vi "save_to_logfile.vi"(0 "file":string, 1 "header_data":string, 3 "to logfile":string[](array[string]), 4 "SAVE":bool, 6 "path":path) -> (10 "writing":bool, 18 "bytes":i64=2275764 format="%.1p")   [LabVIEW 2017, in "ZBOX_IS.lvlib"]
uses:
  ZBOX_IS.lvlib
panel:
  in  "write rate, s":dbl=1.0 min=0.1 max=10.0 step=0.1 format="%#_13g"
  out "to collect":i32=1500
  in  "clear":bool
  out "t write":dbl=3547614984.042773
  in  "DATA RATE, s":dbl=0.001 min=0.001 max=10.0 step=0.001 format="%#_6f"
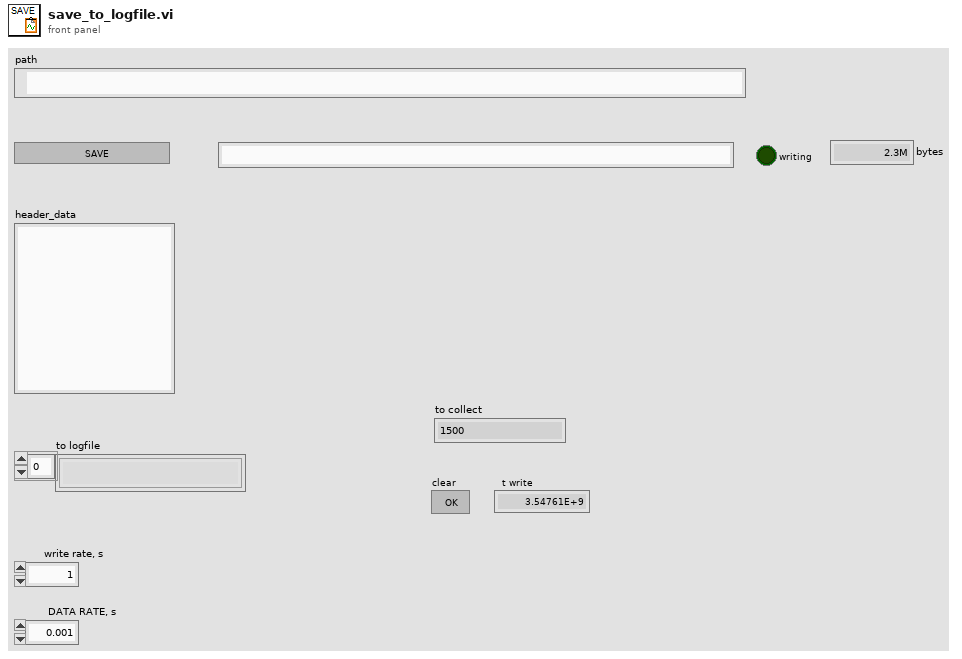
[diagram p1: front panel]
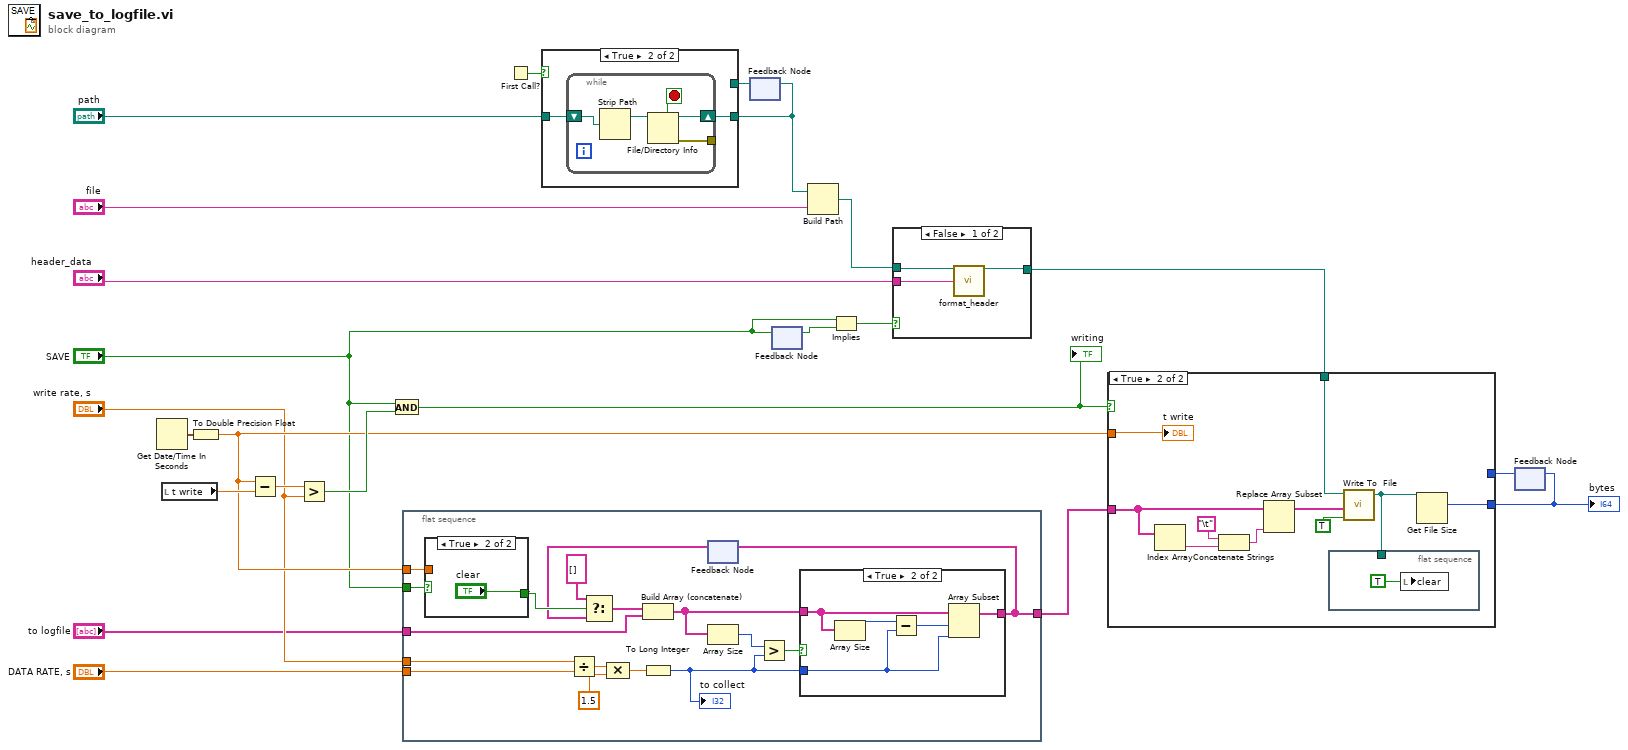
[diagram p0: block diagram]
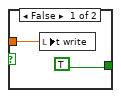
[diagram p3: hidden frame]
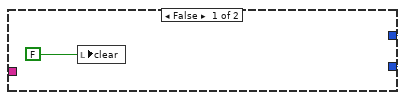
[diagram p6: hidden frame]
diagram:
  n1 = Get Date/Time In Seconds() -> (seconds since 1Jan1904=w21:timestamp)
  n2 = local read "t write"() -> (w22:dbl)
  n3 = To Double Precision Float(number=w21) -> (double precision float=w18:dbl)
  n4 = Subtract(x=w18, y=w22) -> (x-y=w20:dbl)
  n5 = Greater?(x=w20, y="write rate, s") -> (0:w19:bool)
  n6 = And(x="SAVE", y=w19) -> (x .and. y?=w15:bool)
  "writing" <- w15
  n7 = flat-sequence {
    tunnel: "DATA RATE, s" -> [w40]
    tunnel: w18 -> [w39]
    tunnel: "write rate, s" -> [w38]
    tunnel: "SAVE" -> [w37]
    tunnel: "to logfile" -> [w36]
    tunnel: [w34] -> w2
    frame #0 {
      n8 = case shown="True" w37 {
        tunnel: [TRUE ("clear") "clear"] -> w35
        tunnel: w39 -> [w47 _]
        frame False {
          n9 = local write "t write"(w47) -> ()
        }
        frame True {
        }
      }
      n10 = Divide(x=w38, y=w40) -> (x/y=w31:dbl)
      n11 = Compound Arithmetic op=MULTIPLY(w31, 1.5 ("value")) -> (w32:dbl)
      n12 = To Long Integer(number=w32) -> (32bit integer=w30:i32)
      "to collect" <- w30
      n13 = feedback #1() -> (w27:string[])  [unwired: 1 out]
      n14 = Select(t=string[] [], s=w35, f=w27) -> (s? t:f=w24:string[])
      n15 = Build Array (concatenate)(w24, w36) -> (w26:string[])
      n16 = Array Size(array=w26) -> (size(s)=w29:i32)
      n17 = Greater?(x=w29, y=w30) -> (0:w28:bool)
      n18 = case shown="True" w28 {
        tunnel: w26 -> [w41 w46]
        tunnel: [w41 w45] -> w34
        tunnel: w30 -> [_ w43]
        frame False {
        }
        frame True {
          n19 = Array Size(array=w46) -> (size(s)=w42:i32)
          n20 = Subtract(x=w42, y=w43) -> (x-y=w44:i32)
          n21 = Array Subset(array=w46, index=w44, length=w43) -> (w45:string[])
        }
      }
      n22 = feedback-in #1(w34) -> ()
    }
  }
  n23 = First Call?() -> (First Call?: T/F=w9:bool)
  n24 = feedback #2() -> (w6:path)  [unwired: 1 in]
  n25 = case shown="True" w9 {
    tunnel: [w50 w52] -> w7
    tunnel: "path" -> [_ w51]
    tunnel: w6 -> [w50 _]
    frame False {
    }
    frame True {
      n26 = while {
        shift-right: [w54] -> w52
        shift-left: w51 -> [w57]
        tunnel: [w53] -> _
        stop <- w55 stop-if-true
        n27 = Strip Path(path=w57) -> (stripped path=w56:path)  [unwired: 1 out]
        n28 = File/Directory Info(path=w56) -> (path out=w54:path, directory=w55:bool, error out=w53:errorcluster)  [unwired: 1 in, 4 out]
      }
    }
  }
  n29 = feedback-in #2(w7) -> ()
  n30 = feedback #3() -> (w5:bool)  [unwired: 1 out]
  n31 = feedback-in #3("SAVE") -> ()
  n32 = Build Path(base path=w7, name or relative path="file") -> (appended path=w11:path)
  n33 = Implies(1:w5, 2:"SAVE") -> (0:w4:bool)
  n34 = case shown="False" w4 {
    tunnel: [w59 w61] -> w17
    tunnel: w11 -> [w60 w61]
    tunnel: "header_data" -> [w58 _]
    frame False {
      n35 = call "format_header.vi"("file path (dialog if empty)"=w60, "values"=w58) -> ("new file path (Not A Path if cancelled)"=w59:path)  [unwired: 13 in]
    }
    frame True {
    }
  }
  n36 = feedback #4() -> (w12:i64)  [unwired: 1 in]
  n37 = case shown="True" w15 {
    tunnel: w18 -> [_ w73]
    tunnel: w17 -> [_ w71]
    tunnel: [w62 w72] -> w13
    tunnel: w12 -> [w62 _]
    tunnel: w2 -> [_ w68]
    frame False {
      n38 = local write "clear"(FALSE ("clear")) -> ()
    }
    frame True {
      n39 = Index Array(array=w68) -> (element=w67:string)  [unwired: 1 in]
      n40 = Concatenate Strings("\t", w67) -> (w65:string)
      n41 = Replace Array Subset(array=w68, new element=w65) -> (w69:string[])  [unwired: 1 in]
      n42 = flat-sequence {
        tunnel: w64 -> [_]
        frame #0 {
          n43 = local write "clear"(TRUE ("clear")) -> ()
        }
      }
      n44 = call "Write To  File.vi"("append to file? (new file:F)"=TRUE, "1D data"=w69, "file path (dialog if empty)"=w71) -> ("new file path (Not A Path if cancelled)"=w64:path)  [unwired: 5 in]
      n45 = Get File Size(file=w64) -> (size (in bytes)=w72:i64)  [unwired: 1 in, 2 out]
      "t write" <- w73
    }
  }
  "bytes" <- w13
  n46 = feedback-in #4(w13) -> ()
